vi "Handle Error.vi"(8 "error in (no error)":errorcluster, 11 "Freezer in":refnum<class "Freezer.lvclass">) -> (0 "error out":errorcluster, 2 "stop actor?":bool=TRUE, 3 "Freezer out":refnum<class "Freezer.lvclass">)   [LabVIEW 2015, in "cRIO-Carbondioxide.lvlib" / "CO2-Actor.lvlib" / "Freezer.lvclass"]
doc: "(<B>Filename</B>: Actor Framework.lvlib:Actor.lvclass:Handle Error.vi)\n\nDefines how the actor handles an error that occurred while processing a message.\n\nBy default, this method does nothing except stop the actor. This method also treats error code 43 (coming from <B>error in</B>) as a sign that the actor shut down normally. In this situation, the Handle Error method does not return the error on <B>error out</B>, meaning the actor's caller will not receive it. All other error codes will be returned on <B>error out</B>.\n\nA descendant class may override this method to change this behavior."
uses:
  Freezer.lvclass
  CO2 Actor/CO2 Actor.lvclass/CO2 Actor.ctl
  cRIO-CO2 Messages/Log Error Msg/Log Error Msg.lvclass/Log Error Msg.ctl
  <vilib>/ActorFramework/Message Enqueuer/Message Enqueuer.lvclass/Message Enqueuer.ctl
  <vilib>/ActorFramework/Message Enqueuer/Enqueue.vi
  <vilib>/ActorFramework/Message Priority Queue/Priority Enqueue.vi
  cRIO-CO2 Messages/Log Error Msg/Log Error Msg.lvclass
  CO2 Actor/CO2 Actor.lvclass
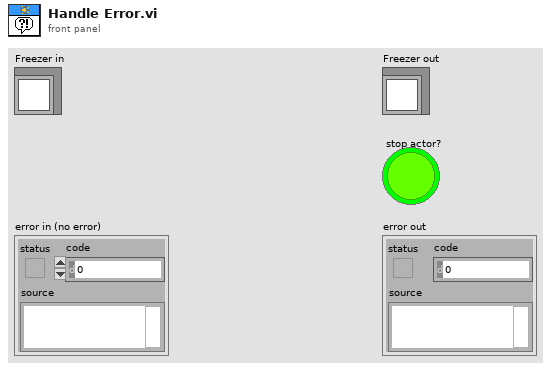
[diagram p1: front panel]
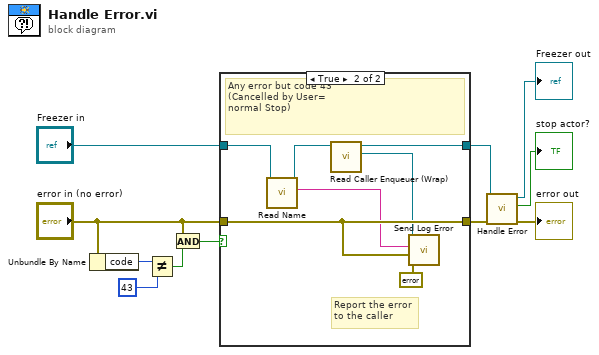
[diagram p0: block diagram]
diagram:
  n1 = Unbundle By Name("error in (no error)") -> ("code"=w7:i32)
  n2 = Not Equal?(x=w7, y=43) -> (x != y?=w5:bool)
  n3 = And(x="error in (no error)", y=w5) -> (x .and. y?=w8:bool)
  n4 = case shown="True" w8 {
    tunnel: "Freezer in" -> [w13 w16]
    tunnel: [w13 w14] -> w1
    tunnel: [w12 w19] -> w3
    tunnel: "error in (no error)" -> [w12 w19]
    frame False {
    }
    frame True {
      # "Report the error\nto the caller"
      # "Any error but code 43\n(Cancelled by User=\nnormal Stop)"
      n5 = call "Read Name.vi"("CO2 Actor in"=w16) -> ("Name"=w18:string, "CO2 Actor out"=w15:refnum<class "Freezer.lvclass">)  [unwired: 9 in]
      n6 = call "Read Caller Enqueuer (Wrap).vi"("CO2 Actor in"=w15) -> ("Actor Framework:Message Enqueuer"=w17:refnum<class "Message Enqueuer.lvclass">, "CO2 Actor out"=w14:refnum<class "Freezer.lvclass">)  [unwired: 9 in]
      n7 = call "Send Log Error.vi"("error in (no error)"=errorcluster {"status"=FALSE, "code"=0, "source"=""}, "error to log (no error)"=w19, "Source Name"=w18, "Message Enqueuer"=w17) -> ()  [unwired: 6 in, 2 out]
    }
  }
  n8 = call-parent "Handle Error.vi"("error in (no error)"=w3, "CO2 Actor in"=w1) -> ("error out"=→"error out":errorcluster, "stop actor?"=→"stop actor?":bool, "CO2 Actor out"=→"Freezer out":refnum<class "Freezer.lvclass">)  [unwired: 7 in]
